vi "createSelfReference.vi"(8 "error in (no error)":errorcluster, 11 "Connection in":refnum<class "Connection.lvclass">) -> (0 "error out":errorcluster, 3 "Connection out":refnum<class "Connection.lvclass">)   [LabVIEW 2013, in "MQTT_Connection.lvlib" / "Connection.lvclass"]
uses:
  Connection.lvclass
  connection event -- cluster.ctl
  Connection.lvclass/Connection.ctl
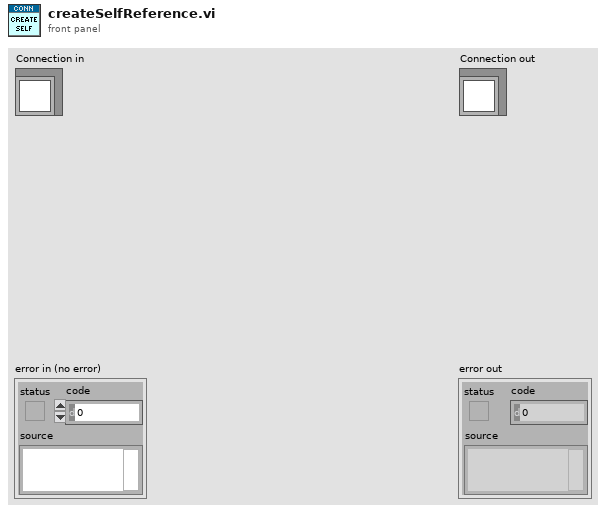
[diagram p1: front panel]
types:
  T1 = typedef "MQTT_Connection.lvlib/Connection.lvclass/connection event -- cluster.ctl" = cluster{"connected":bool, "reason":i32}
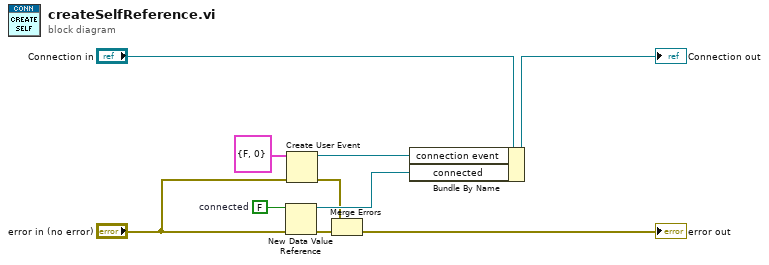
[diagram p0: block diagram]
diagram:
  w8 = FALSE  # connected
  n1 = New Data Value Reference(data value=w8, error in="error in (no error)") -> (data value reference=w7:refnum<data-value>, error out=w2:errorcluster)
  n2 = Create User Event(user event datatype=T1 {"connected"=FALSE, "reason"=0} ("Connection event"), error in="error in (no error)") -> (user event=w5:refnum<user-event>, error out=w3:errorcluster)
  n3 = Merge Errors(w3, w2) -> (→"error out":errorcluster)
  n4 = Bundle By Name(cluster="Connection in", "connection event"=w5, "connected"=w7) -> (→"Connection out":refnum<class "Connection.lvclass">)
